vi "DFConfig Get Tagged Section.vi"(8 "Replacement String (\"\")":string, 10 "Tag (\"\")":string, 11 "String":string) -> (0 "String with Replacement":string, 1 "End Tag":string, 2 "Start Tag":string, 4 "Not Found?":bool, 5 "InnerString":string)   [LabVIEW 2011]
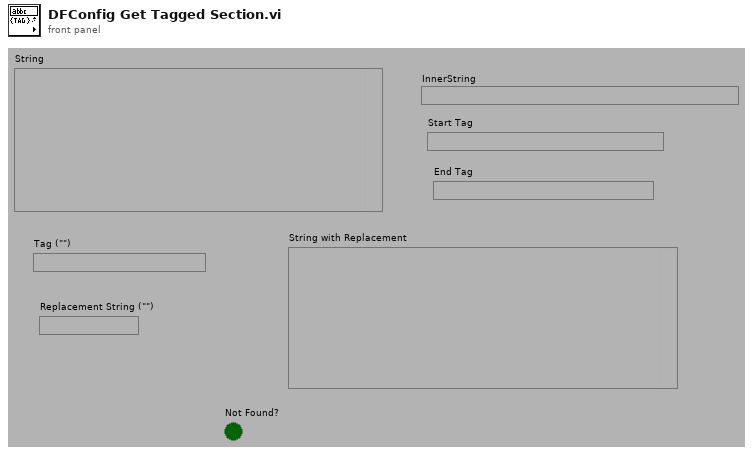
[diagram p1: front panel]
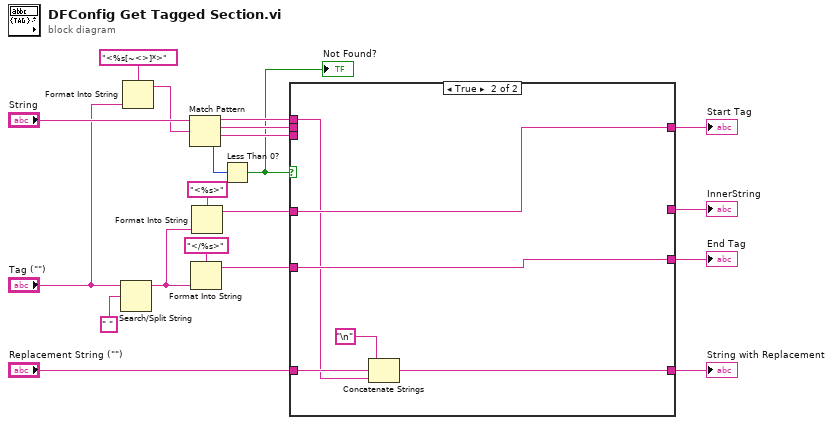
[diagram p0: block diagram]
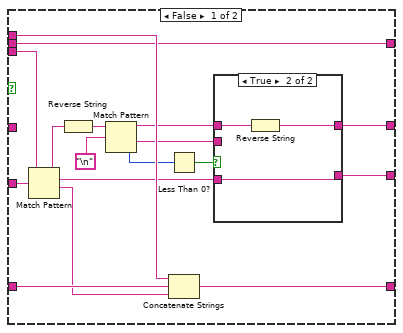
[diagram p2: hidden frame]
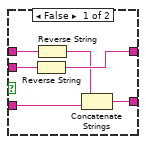
[diagram p3: hidden frame]
diagram:
  n1 = Search/Split String(string="Tag (\"\")", search string/char (-)=" ") -> (substring before match=w1:string)  [unwired: 3 out]
  n2 = Format Into String(format string="<%s[~<>]*>", "Tag (\"\")") -> (resulting string=w13:string)  [unwired: 2 in, 1 out]
  n3 = Match Pattern(string="String", regular expression=w13) -> (before substring=w18:string, match substring=w8:string, after substring=w19:string, offset past match=w9:i32)  [unwired: 1 out]
  n4 = Format Into String(format string="</%s>", w1) -> (resulting string=w14:string)  [unwired: 2 in, 1 out]
  n5 = Format Into String(format string="<%s>", w1) -> (resulting string=w2:string)  [unwired: 2 in, 1 out]
  n6 = Less Than 0?(x=w9) -> (x < 0?=w6:bool)
  "Not Found?" <- w6
  n7 = case shown="True" w6 {
    tunnel: w19 -> [w37 _]
    tunnel: w18 -> [w36 w49]
    tunnel: [w25 w48] -> w17
    tunnel: w14 -> [w35 w52]
    tunnel: "Replacement String (\"\")" -> [w34 w50]
    tunnel: [w29 w52] -> w11
    tunnel: [w23 _] -> w10
    tunnel: w8 -> [w27 _]
    tunnel: [w27 w51] -> w7
    tunnel: w2 -> [_ w51]
    frame False {
      n8 = Match Pattern(string=w37, regular expression=w35) -> (before substring=w33:string, match substring=w30:string, after substring=w26:string)  [unwired: 2 out]
      n9 = Reverse String(1:w33) -> (0:w24:string)
      n10 = Match Pattern(string=w24, regular expression="\n") -> (before substring=w28:string, after substring=w31:string, offset past match=w22:i32)  [unwired: 2 out]
      n11 = Less Than 0?(x=w22) -> (x < 0?=w21:bool)
      n12 = Concatenate Strings(w36, w34, w26) -> (w25:string)
      n13 = case shown="True" w21 {
        tunnel: w31 -> [w43 _]
        tunnel: w30 -> [w42 w44]
        tunnel: [w41 w44] -> w29
        tunnel: w28 -> [w40 w46]
        tunnel: [w39 w45] -> w23
        frame False {
          n14 = Reverse String(1:w43) -> (0:w39:string)
          n15 = Reverse String(1:w40) -> (0:w38:string)
          n16 = Concatenate Strings(w38, w42) -> (w41:string)
        }
        frame True {
          n17 = Reverse String(1:w46) -> (0:w45:string)
        }
      }
    }
    frame True {
      n18 = Concatenate Strings("\n", w50, w49) -> (w48:string)
    }
  }
  "String with Replacement" <- w17
  "InnerString" <- w10
  "End Tag" <- w11
  "Start Tag" <- w7
